vi "goto_point.vi"(2 "rev":bool, 3 "direction":dbl, 4 "distance":dbl) -> (0 "R":i16, 1 "L":i16)   [LabVIEW 2013]
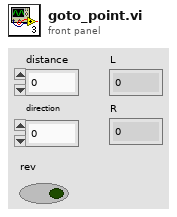
[diagram p1: front panel]
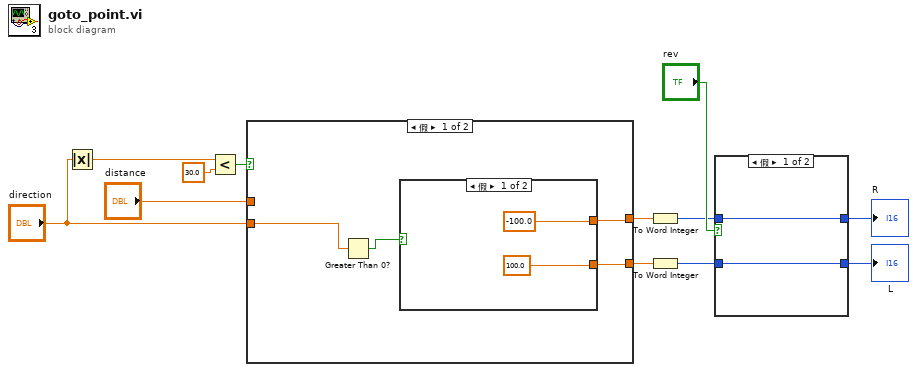
[diagram p0: block diagram]
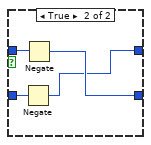
[diagram p2: hidden frame]
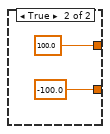
[diagram p3: hidden frame]
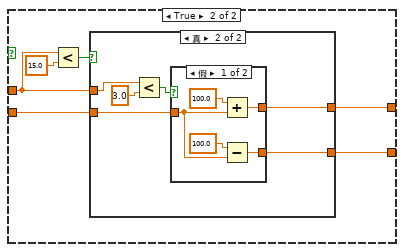
[diagram p4: hidden frame]
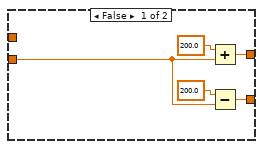
[diagram p5: hidden frame]
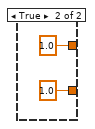
[diagram p6: hidden frame]
diagram:
  n1 = Absolute Value(x="direction") -> (abs(x)=w9:dbl)
  n2 = Less?(x=w9, y=30.0) -> (x < y?=w7:bool)
  n3 = case shown="假" w7 {
    tunnel: [w14 w23] -> w11
    tunnel: [w13 w22] -> w10
    tunnel: "direction" -> [w16 w24]
    tunnel: "distance" -> [_ w21]
    frame False {
      n4 = Greater Than 0?(x=w16) -> (x > 0?=w15:bool)
      n5 = case shown="假" w15 {
        tunnel: [-100.0 100.0] -> w14
        tunnel: [100.0 -100.0] -> w13
        frame False {
        }
        frame True {
        }
      }
    }
    frame True {
      n6 = Less?(x=w21, y=15.0) -> (x < y?=w25:bool)
      n7 = case shown="真" w25 {
        tunnel: w24 -> [w31 w37]
        tunnel: [w28 w33] -> w23
        tunnel: [w27 w32] -> w22
        tunnel: w21 -> [_ w35]
        frame False {
          n8 = Add(x=200.0, y=w31) -> (x+y=w28:dbl)
          n9 = Subtract(x=200.0, y=w31) -> (x-y=w27:dbl)
        }
        frame True {
          n10 = Less?(x=w35, y=3.0) -> (x < y?=w36:bool)
          n11 = case shown="假" w36 {
            tunnel: w37 -> [w40 _]
            tunnel: [w39 1.0] -> w33
            tunnel: [w38 1.0] -> w32
            frame False {
              n12 = Add(x=100.0, y=w40) -> (x+y=w39:dbl)
              n13 = Subtract(x=100.0, y=w40) -> (x-y=w38:dbl)
            }
            frame True {
            }
          }
        }
      }
    }
  }
  n14 = To Word Integer(number=w11) -> (16bit integer=w4:i16)
  n15 = To Word Integer(number=w10) -> (16bit integer=w2:i16)
  n16 = case shown="假" "rev" {
    tunnel: [w46 w47] -> w3
    tunnel: w4 -> [w46 w50]
    tunnel: [w45 w49] -> w1
    tunnel: w2 -> [w45 w48]
    frame False {
    }
    frame True {
      n17 = Negate(x=w48) -> (-x=w47:i16)
      n18 = Negate(x=w50) -> (-x=w49:i16)
    }
  }
  "R" <- w3
  "L" <- w1
